vi "test_TxUDP-RxUDP.vi"(8 "error in":errorcluster, 11 "reference in":refnum<class "AIM ARINC 664 Loopback.lvclass">) -> (0 "error out":errorcluster, 3 "reference out":refnum<class "AIM ARINC 664 Loopback.lvclass">)   [LabVIEW 2020, in "AIM ARINC 664 Loopback.lvclass"]
uses:
  AIM ARINC 664 Loopback.lvclass
  AIM ARINC 664 Loopback.lvclass/AIM ARINC 664 Loopback.ctl
  <vilib>/addons/_JKI Toolkits/VI Tester/TestCase.llb/TestCase.lvclass
  6a3dd3ed-914d-4d14-bf18-724521aa5e28.vi
  NationalInstruments.VeriStand.SystemDefinitionAPI
  Scripting/AIM ARINC 664 Scripting.lvlib
  Import/AIM ARINC 664 Import.lvlib
  <vilib>/NI/VeriStand Custom Device Testing Tools/VeriStandTestCase/VeriStandTestCase.lvclass
  8abe1e9f-12f7-4d29-bb0e-ea5e1950c3f4.vi
  b47c41b5-a02e-49d5-b852-4e28f097d7ad.vi
panel:
  out "resulting string":string
  # "This test is disabled fro now because the configuration is between two cards. If \nyou need to setup this, change from the two cards to one card configuration as below:"
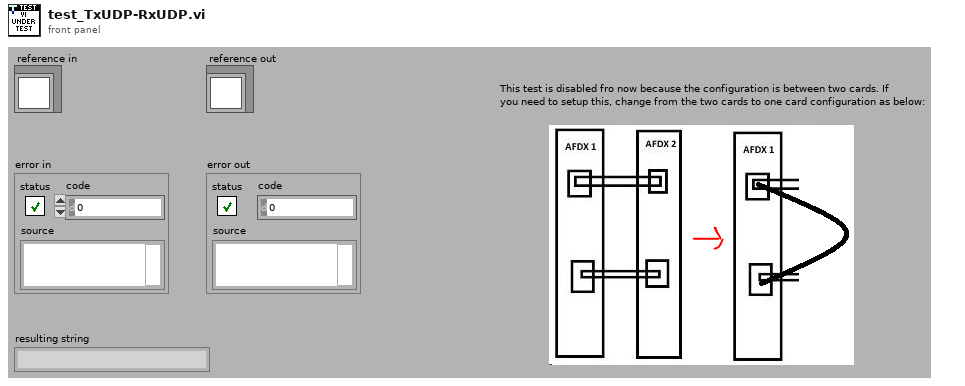
[diagram p1: front panel]
types:
  T1 = typedef "Custom Device API.lvlib/Custom Device Item Ref.ctl" = u64
  T2 = typedef "AIM ARINC 664 Import.lvlib/Board Top Level Configuration.ctl" = cluster{"boardSetup":T3, "portConfiguration":T4[]}
  T3 = typedef "AIM ARINC 664 Import.lvlib/board_setup.ctl" = cluster{"boardId":u32, "portSpeed":u32, "portConfig":u32}
  T4 = typedef "AIM ARINC 664 Import.lvlib/port_configuration.ctl" = cluster{"portSetup":T5, "Tx_Generic":T6[], "Rx_Monitor":cluster{"DefaultCronoMode":u32, "GlbMonBufferSizeIn":u32, "CaptureMode":u32, "MaxFileSizeMB":u32, "Strobe":u32, "TriggerPosition":u32}[], "Tx_UDP":cluster{"tx_udp_setup":cluster{"VlId":i32, "Bag":i32, "NetSelect":u32, "domainID":u8, "sideID":u8, "locationID":u8, "interfaceID":u8, "NumOfSubVl":u16, "Skew":u32, "MaxFrameLength":u32, "FrameBufferSize":u32}, "commPorts":T14[], "sapPorts":T15[]}[], "Rx_UDP":cluster{"Tx_UDP":T16, "commPorts":T17[], "sapPorts":T18[]}[]}
  T5 = typedef "AIM ARINC 664 Import.lvlib/port_setup.ctl" = cluster{"port Id":u32, "redundant":bool}
  T6 = typedef "AIM ARINC 664 Import.lvlib/session_tx_generic.ctl" = cluster{"tx_generic_setup":T7, "Frame Headers":T8[]}
  T7 = typedef "AIM ARINC 664 Import.lvlib/tx_generic_setup.ctl" = cluster{"QueueSizeIn":u32, "Count":i32, "StartMode":i32}
  T8 = typedef "AIM ARINC 664 Import.lvlib/frame_tx_generic.ctl" = cluster{"FrameID":string, "PayloadID":string, "Frame header":cluster{"FrameStartMode":i32, "InterFrameGap":i32, "PacketGroupWaitTime":i32, "NetSelect":u32, "PayloadBufferMode":i32, "PayloadGenerationMode":i32, "PhysErrorInjection":i32, "PreambleCount":i32, "SequenceNumberInit":T9, "SequenceNumberOffset":T10, "Skew":i32}, "Parameters":T11[]}
  T9 = typedef "AIM ARINC 664 Import.lvlib/frame_tx_generic_seqNumberInit.ctl" = i32
  T10 = typedef "AIM ARINC 664 Import.lvlib/frame_tx_generic_seqNumberOffset.ctl" = i32
  T11 = typedef "AIM ARINC 664 Import.lvlib/frame_parameter.ctl" = cluster{"name":string, "default value":dbl, "unit":string, "Parameter":T12}
  T12 = typedef "AIM ARINC 664 Import.lvlib/frame_parameter_definition.ctl" = cluster{"start index":i32, "size":i32, "encoding":T13, "signed":bool, "scale multiplier":dbl, "scale offset":dbl}
  T13 = typedef "Encoding (Arinc664).ctl" = u16
  T14 = typedef "AIM ARINC 664 Import.lvlib/port_tx_udp_comm.ctl" = cluster{"PayloadID":string, "partitionID":u8, "UdpSrcPort":u16, "UdpDstPort":u16, "PortType":enum16{"FDX_UDP_SAMPLING", "FDX_UDP_QUEUING"}, "SubVIId":u32, "UdpNumBufMessages":u32, "UdpMaxMessageSize":u32, "UdpSamplingRate":u32, "Parameters":T11[]}
  T15 = typedef "AIM ARINC 664 Import.lvlib/port_tx_udp_sap.ctl" = cluster{"PayloadID":string, "SubVlId":u8, "UdpSrcPort":u16, "UdpNumBufMessages":u32, "UdpMaxMessageSize":u32, "partitionID":u8, "domainID":u8, "sideID":u8, "locationID":u8, "interfaceID":u8, "Parameters":T11[]}
  T16 = typedef "AIM ARINC 664 Import.lvlib/rx_udp_setup.ctl" = cluster{"VerificationMode":u32, "Bag":u32, "Jitter":u32, "MaxFrameLength":u32, "MaxSkew":u32, "VLBufSize":u32, "FilterMode":u32, "FilterPosition":u32, "Padding":u32, "FilterMask":u32, "FilterData":u32, "MinFrameLength":u32, "VlId":u16, "VLRange":u32}
  T17 = typedef "AIM ARINC 664 Import.lvlib/port_rx_udp_comm.ctl" = cluster{"PayloadID":string, "domainID":u8, "sideID":u8, "locationID":u8, "partitionID":u8, "UdpSrcPort":u16, "UdpDstPort":u16, "PortType":enum16{"FDX_UDP_SAMPLING", "FDX_UDP_QUEUING"}, "SubVIId":u32, "UdpNumBufMessages":u32, "UdpMaxMessageSize":u32, "UdpSamplingRate":u32, "Parameters":T11[]}
  T18 = typedef "AIM ARINC 664 Import.lvlib/port_rx_udp_sap.ctl" = cluster{"PayloadID":string, "UdpDstPort":u16, "UdpNumBufMessages":u32, "UdpMaxMessageSize":u32, "Parameters":T11[]}
  T19 = typedef "Payload Map.ctl" = map{string, T20}
  T20 = typedef "Payload Record Type.ctl" = cluster{"Data":u8[], "Type of Frame":T21}
  T21 = typedef "Type of Payload.ctl" = u16
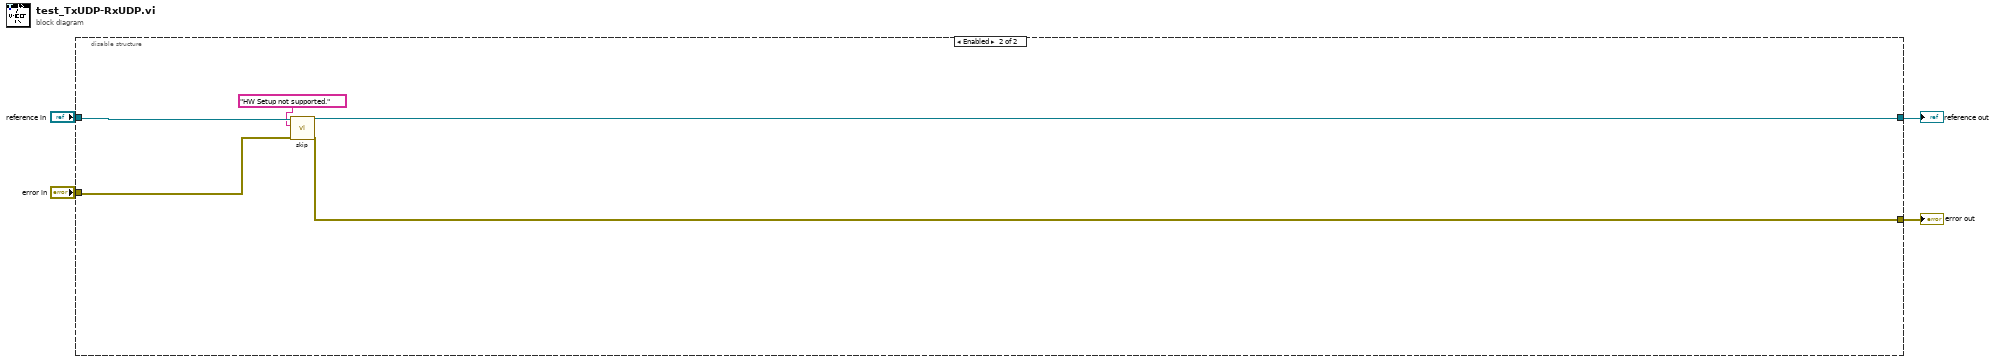
[diagram p0: block diagram]
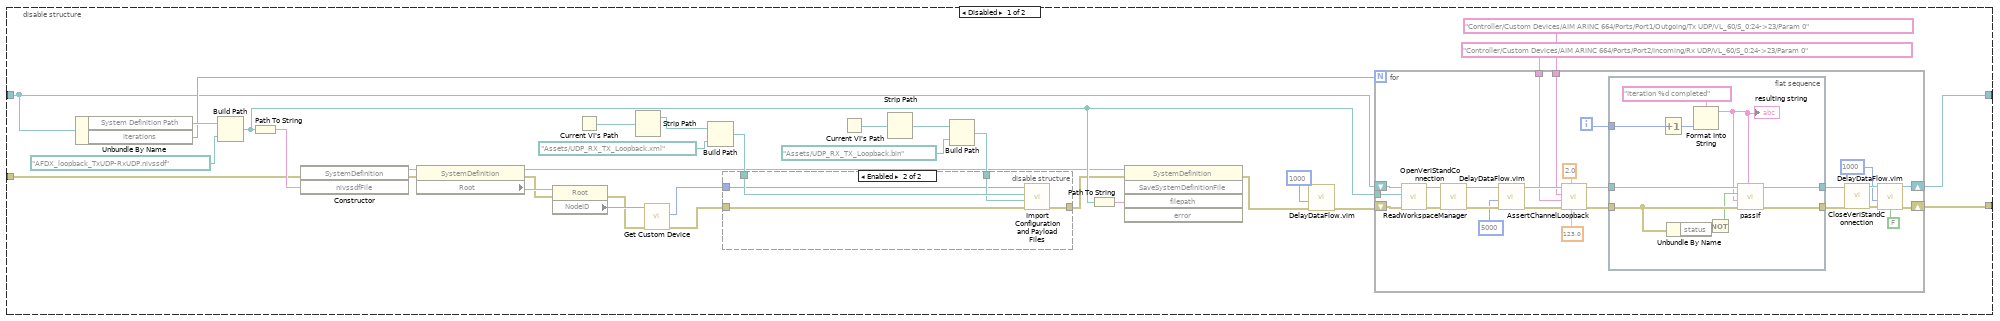
[diagram p2: hidden frame]
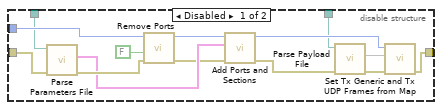
[diagram p3: hidden frame]
diagram:
  n1 = disable-structure shown="Enabled" {
    disable-tunnel: "reference in" -> [w5 w94]
    disable-tunnel: "error in" -> [w6 w93]
    disable-tunnel: [w35 w92] -> w2
    disable-tunnel: [w34 w91] -> w1
    frame Disabled {
      n2 = Unbundle By Name(w5) -> ("System Definition Path"=w37:path, "iterations"=w12:i32)
      n3 = Build Path(base path=w37, name or relative path=path "AFDX_loopback_TxUDP-RxUDP.nivssdf") -> (appended path=w32:path)
      n4 = Path To String(path=w32) -> (string=w33:string)
      n5 = constructor class="SystemDefinition"(error in=w6, "nivssdfFile"=w33) -> (reference out=w31:refnum<k24>, error out=w29:errorcluster)  [unwired: 2 in, 2 out]
      n6 = property class="SystemDefinition"(reference=w31, error in=w29) -> (reference out=w18:refnum<k24>, error out=w28:errorcluster, "Root"=w30:refnum<k24>)
      n7 = property class="Root"(reference=w30, error in=w28) -> (error out=w15:errorcluster, "NodeID"=w16:u64)  [unwired: 1 out]
      n8 = Current VI's Path() -> (path=w27:path)
      n9 = Strip Path(path=w27) -> (stripped path=w21:path)  [unwired: 1 out]
      n10 = call "Get Custom Device.vi"("error in"=w15, "custom device ref in"=w16) -> ("error out"=w14:errorcluster, "First Item Ref"=w13:T1)  [unwired: 5 in, 3 out]
      n11 = Build Path(base path=w21, name or relative path=path "Assets/UDP_RX_TX_Loopback.xml") -> (appended path=w22:path)
      n12 = Current VI's Path() -> (path=w25:path)
      n13 = Strip Path(path=w25) -> (stripped path=w20:path)  [unwired: 1 out]
      n14 = Build Path(base path=w20, name or relative path=path "Assets/UDP_RX_TX_Loopback.bin") -> (appended path=w23:path)
      n15 = disable-structure shown="Enabled" {
        disable-tunnel: w13 -> [w83 w85]
        disable-tunnel: w14 -> [w75 w89]
        disable-tunnel: w23 -> [w73 w86]
        disable-tunnel: w22 -> [w72 w87]
        disable-tunnel: [w71 w88] -> w19
        frame Disabled {
          n16 = call "Parse Parameters File.vi"("error in"=w75, "path to XML document"=w72) -> ("error out"=w84:errorcluster, "board configuration out"=w81:T2)  [unwired: 7 in, 1 out]
          n17 = call "Remove Ports.vi"("error in"=w84, "refresh?"=FALSE, "Custom device Ref"=w83) -> ("error out"=w80:errorcluster, "Custom device Ref out"=w82:T1)  [unwired: 7 in]
          n18 = call "Add Ports and Sections.vi"("error in"=w80, "board configuration in"=w81, "custom device ref"=w82) -> ("error out"=w79:errorcluster, "custom device ref out"=w74:T1)  [unwired: 7 in]
          n19 = call "Parse Payload File.vi"("error in"=w79, "frame array path in"=w73) -> ("error out"=w78:errorcluster, "Map"=w77:T19)  [unwired: 7 in, 1 out]
          n20 = call "Set Tx Generic and Tx UDP Frames from Map.vi"("error in"=w78, "payload map"=w77, "custom device ref"=w74) -> ("error out"=w71:errorcluster)  [unwired: 7 in, 1 out]
        }
        frame Enabled {
          n21 = call "Import Configuration and Payload Files.vi"("error in"=w89, "payload file path"=w86, "parameters configuration file path"=w87, "custom device ref"=w85) -> ("error out"=w88:errorcluster)  [unwired: 6 in, 1 out]
        }
      }
      n22 = Path To String(path=w32) -> (string=w17:string)
      n23 = invoke class="SystemDefinition" method="SaveSystemDefinitionFile"(reference=w18, error in=w19, "filepath"=w17) -> (error out=w11:errorcluster)  [unwired: 2 in, 4 out]
      n24 = call "DelayDataFlow.vim"("value in"=w11, "milliseconds to wait"=u32 1000) -> ("value out"=w10:errorcluster)  [unwired: 2 in, 1 out]
      n25 = for {
        N: w12 -> [_]
        tunnel: w32 -> [w53]
        shift-right: [w58] -> w34
        shift-left: w5 -> [w60]
        shift-right: [w47] -> w35
        shift-left: w10 -> [w54]
        tunnel: "Controller/Custom Devices/AIM ARINC 664/Ports/Port2/Incoming/Rx UDP/VL_60/S_0:24->23/Param 0" -> [w39]
        tunnel: "Controller/Custom Devices/AIM ARINC 664/Ports/Port1/Outgoing/Tx UDP/VL_60/S_0:24->23/Param 0" -> [w38]
        i -> [w41]
        n26 = call-dynamic "OpenVeriStandConnection.vi"("error in (no error)"=w54, "System Definition File"=w53, "VeriStand Test Case in"=w60) -> ("error out"=w59:errorcluster, "VeriStand Test Case out"=w57:refnum<class "AIM ARINC 664 Loopback.lvclass">)  [unwired: 6 in, 1 out]
        n27 = call-dynamic "ReadWorkspaceManager.vi"("error in (no error)"=w59, "VeriStand Test Case in"=w57) -> ("error out"=w56:errorcluster, "VeriStand Test Case out"=w51:refnum<class "AIM ARINC 664 Loopback.lvclass">)  [unwired: 7 in, 1 out]
        n28 = call "DelayDataFlow.vim"("value in"=w56, "milliseconds to wait"=u32 5000) -> ("value out"=w52:errorcluster)  [unwired: 2 in, 1 out]
        n29 = call <vilib>:"AssertChannelLoopback.vi"("Value"=123.0, "Timeout (1 second)"=2.0, "error in (no error)"=w52, "Read Channel"=w39, "Write Channel"=w38, "VeriStand Test Case in"=w51) -> ("error out"=w42:errorcluster, "VeriStand Test Case out"=w40:refnum<class "AIM ARINC 664 Loopback.lvclass">)  [unwired: 4 in]
        n30 = flat-sequence {
          tunnel: [w70] -> w44
          tunnel: [w69] -> w43
          tunnel: w42 -> [w68]
          tunnel: w41 -> [w64]
          tunnel: w40 -> [w62]
          frame #0 {
            n31 = Increment(x=w64) -> (x+1=w63:i32)
            n32 = Unbundle By Name(w68) -> ("status"=w67:bool)
            n33 = Format Into String(format string="Iteration %d completed", w63) -> (resulting string=w61:string)  [unwired: 2 in, 1 out]
            "resulting string" <- w61
            n34 = Not(x=w67) -> (.not. x?=w66:bool)
            n35 = call-dynamic "passIf.vi"("custom report message (\"\")"=w61, "error in (no error)"=w68, "message (\"\")"=w61, "pass"=w66, "TestCase in"=w62) -> ("error out"=w69:errorcluster, "TestCase out"=w70:refnum<class "AIM ARINC 664 Loopback.lvclass">)  [unwired: 5 in]
          }
        }
        n36 = call-dynamic "CloseVeriStandConnection.vi"("error in (no error)"=w43, "VeriStand Test Case in"=w44) -> ("error out"=w48:errorcluster, "VeriStand Test Case out"=w58:refnum<class "AIM ARINC 664 Loopback.lvclass">)  [unwired: 8 in]
        n37 = call "DelayDataFlow.vim"("value in"=w48, "milliseconds to wait"=u32 1000, "no delay on error (T)"=FALSE) -> ("value out"=w47:errorcluster)  [unwired: 1 in, 1 out]
      }
    }
    frame Enabled {
      n38 = call <vilib>:"skip.vi"("error in (no error)"=w93, "skipMessage"="HW Setup not supported.", "TestCase in"=w94) -> ("error out"=w92:errorcluster, "TestCase out"=w91:refnum<class "AIM ARINC 664 Loopback.lvclass">)  [unwired: 7 in]
    }
  }
  "error out" <- w2
  "reference out" <- w1
